vi "getFrameFormat.vi"() -> ()   [LabVIEW 2012]
uses:
  hidapi_32bits.dll
panel:
  out "return type":i32
  out "numOfPixelsInFrame":u16[](array[numeric])
  out "reductionMode":u8[](array[numeric])
  out "numOfEndElement":u16[](array[numeric])
  out "numOfStartElement":u16[](array[numeric])
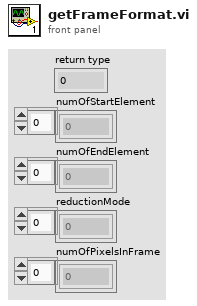
[diagram p1: front panel]
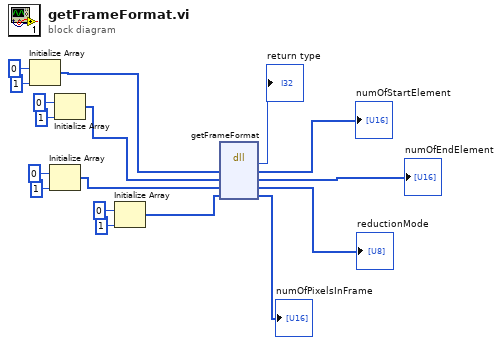
[diagram p0: block diagram]
diagram:
  n1 = Initialize Array(u16 0 ("element"), 1 ("dimension size")) -> (w17:u16[])
  n2 = Initialize Array(u16 0 ("element"), 1 ("dimension size")) -> (w8:u16[])
  n3 = Initialize Array(u16 0 ("element"), 1 ("dimension size")) -> (w11:u16[])
  n4 = Initialize Array(u16 0 ("element"), 1 ("dimension size")) -> (w5:u16[])
  n5 = dll-call lib="C:/All_Data/mikrocont/Project1/New_controller__Jan_2015/LabView_Aug_2015/hidapi_32bits.dll" fn="getFrameFormat"("numOfStartElement"=w17, "numOfEndElement"=w11, "reductionMode"=w8, "numOfPixelsInFrame"=w5) -> ("return type"=→"return type":i32, "numOfStartElement"=→"numOfStartElement":u16[], "numOfEndElement"=→"numOfEndElement":u16[], "reductionMode"=→"reductionMode":u8[], "numOfPixelsInFrame"=→"numOfPixelsInFrame":u16[])  [unwired: 3 in, 2 out]
